vi "CRYASIORemoveInputWave.vi"(8 "OCI":u32, 11 "error in (no error)":errorcluster) -> (0 "bResult":bool, 3 "error out":errorcluster)   [LabVIEW 2013]
uses:
  CRY_ASIO.dll
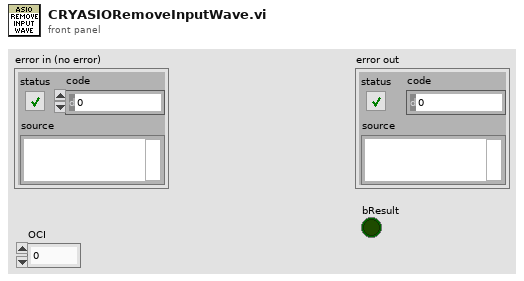
[diagram p1: front panel]
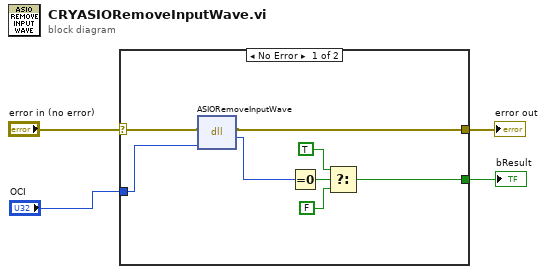
[diagram p0: block diagram]
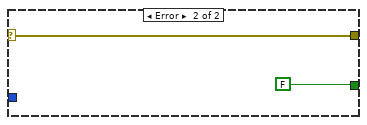
[diagram p2: hidden frame]
diagram:
  n1 = case shown="No Error" "error in (no error)" {
    selector: "error in (no error)" -> [w8 w14]
    tunnel: [w7 w14] -> w3
    tunnel: "OCI" -> [w6 _]
    tunnel: [w9 FALSE] -> w1
    frame No Error {
      n2 = dll-call lib="D:/LabView_Project/CRY6181/CRY_ASIO.dll" fn="ASIORemoveInputWave"(error in=w8, "arg1"=w6) -> (error out=w7:errorcluster, "return type"=w5:u32)  [unwired: 3 in, 1 out]
      n3 = Equal To 0?(x=w5) -> (x = 0?=w12:bool)
      n4 = Select(t=TRUE, s=w12, f=FALSE) -> (s? t:f=w9:bool)
    }
    frame Error {
    }
  }
  "error out" <- w3
  "bResult" <- w1
